vi "To Float Tree Data.vi"(10 "Float":dbl) -> (3 "Float Tree Data":refnum<class "Flt.lvclass">)   [LabVIEW 2017, in "Tree API.lvlib" / "Flt.lvclass"]
doc: "Convert a Float value to Tree Data type."
uses:
  Flt.lvclass
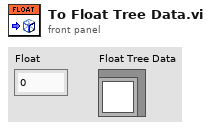
[diagram p1: front panel]
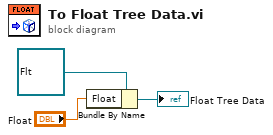
[diagram p0: block diagram]
diagram:
  n1 = Bundle By Name(cluster=refnum<class "Flt.lvclass"> refnum ("Float in"), "Float"="Float") -> (→"Float Tree Data":refnum<class "Flt.lvclass">)
